vi "LogicalSort.vi"(2 "Input Array":cluster{"date/time string":string, i32}[](array[cluster])=[{"date/time string"="NI_ChannelLength", 0}, {"date/time string"="NI_DataType", 1}, {"date/time string"="name", 2}, {"date/time string"="NI_Scaling_Status", 3}, {"date/time string"="NI_Number_Of_Scales", 4}, {"date/time string"="NI_Scale[1]_Scale_Type", 5}, {"date/time string"="NI_Scale[1]_Linear_Slope", 6}, {"date/time string"="NI_Scale[1]_Linear_Y_Intercept", 7}, {"date/time string"="NI_Scale[1]_Linear_Input_Source", 8}, {"date/time string"="NI_Scale[3]_Scale_Type", 9}, {"date/time string"="NI_Scale[3]_Linear_Slope", 10}, {"date/time string"="NI_Scale[3]_Linear_Y_Intercept", 11}, {"date/time string"="NI_Scale[3]_Linear_Input_Source", 12}, {"date/time string"="NI_Scale[4]_Scale_Type", 13}, {"date/time string"="NI_Scale[4]_Subtract_Left_Operand_Input_Source", 14}, {"date/time string"="NI_Scale[4]_Subtract_Right_Operand_Input_Source", 15}, {"date/time string"="NI_Scale[5]_Scale_Type", 16}, {"date/time string"="NI_Scale[5]_Linear_Slope", 17}, {"date/time string"="NI_Scale[5]_Linear_Y_Intercept", 18}, {"date/time string"="NI_Scale[5]_Linear_Input_Source", 19}, {"date/time string"="NI_Scale[7]_Scale_Type", 20}, {"date/time string"="NI_Scale[7]_Linear_Slope", 21}, {"date/time string"="NI_Scale[7]_Linear_Y_Intercept", 22}, {"date/time string"="NI_Scale[7]_Linear_Input_Source", 23}, {"date/time string"="NI_Scale[9]_Scale_Type", 24}, {"date/time string"="NI_Scale[9]_Linear_Slope", 25}, {"date/time string"="NI_Scale[9]_Linear_Y_Intercept", 26}, {"date/time string"="NI_Scale[9]_Linear_Input_Source", 27}, {"date/time string"="NI_Scale[10]_Scale_Type", 28}, {"date/time string"="NI_Scale[10]_Subtract_Left_Operand_Input_Source", 29}, {"date/time string"="NI_Scale[10]_Subtract_Right_Operand_Input_Source", 30}, {"date/time string"="NI_Scale[11]_Scale_Type", 31}, {"date/time string"="NI_Scale[11]_Table_Scaled_Values_Size", 32}, {"date/time string"="NI_Scale[11]_Table_Scaled_Values[0]", 33}, {"date/time string"="NI_Scale[11]_Table_Scaled_Values[1]", 34}, {"date/time string"="NI_Scale[11]_Table_Scaled_Values[2]", 35}, {"date/time string"="NI_Scale[11]_Table_Scaled_Values[3]", 36}, {"date/time string"="NI_Scale[11]_Table_Scaled_Values[4]", 37}, {"date/time string"="NI_Scale[11]_Table_Scaled_Values[5]", 38}, {"date/time string"="NI_Scale[11]_Table_Scaled_Values[6]", 39}, {"date/time string"="NI_Scale[11]_Table_Scaled_Values[7]", 40}, {"date/time string"="NI_Scale[11]_Table_Scaled_Values[8]", 41}, {"date/time string"="NI_Scale[11]_Table_Scaled_Values[9]", 42}, {"date/time string"="NI_Scale[11]_Table_Scaled_Values[10]", 43}, {"date/time string"="NI_Scale[11]_Table_Scaled_Values[11]", 44}, {"date/time string"="NI_Scale[11]_Table_Scaled_Values[12]", 45}, {"date/time string"="NI_Scale[11]_Table_Scaled_Values[13]", 46}, {"date/time string"="NI_Scale[11]_Table_Scaled_Values[14]", 47}, {"date/time string"="NI_Scale[11]_Table_Scaled_Values[15]", 48}, {"date/time string"="NI_Scale[11]_Table_Scaled_Values[16]", 49}, {"date/time string"="NI_Scale[11]_Table_Scaled_Values[17]", 50}, {"date/time string"="NI_Scale[11]_Table_Scaled_Values[18]", 51}, {"date/time string"="NI_Scale[11]_Table_Scaled_Values[19]", 52}, {"date/time string"="NI_Scale[11]_Table_Scaled_Values[20]", 53}, {"date/time string"="NI_Scale[11]_Table_Scaled_Values[21]", 54}, {"date/time string"="NI_Scale[11]_Table_Scaled_Values[22]", 55}, {"date/time string"="NI_Scale[11]_Table_Scaled_Values[23]", 56}, {"date/time string"="NI_Scale[11]_Table_Scaled_Values[24]", 57}, {"date/time string"="NI_Scale[11]_Table_Scaled_Values[25]", 58}, {"date/time string"="NI_Scale[11]_Table_Scaled_Values[26]", 59}, {"date/time string"="NI_Scale[11]_Table_Scaled_Values[27]", 60}, {"date/time string"="NI_Scale[11]_Table_Scaled_Values[28]", 61}, {"date/time string"="NI_Scale[11]_Table_Scaled_Values[29]", 62}, {"date/time string"="NI_Scale[11]_Table_Scaled_Values[30]", 63}, {"date/time string"="NI_Scale[11]_Table_Scaled_Values[31]", 64}, {"date/time string"="NI_Scale[11]_Table_Scaled_Values[32]", 65}, {"date/time string"="NI_Scale[11]_Table_Scaled_Values[33]", 66}, {"date/time string"="NI_Scale[11]_Table_Scaled_Values[34]", 67}, {"date/time string"="NI_Scale[11]_Table_Scaled_Values[35]", 68}, {"date/time string"="NI_Scale[11]_Table_Scaled_Values[36]", 69}, {"date/time string"="NI_Scale[11]_Table_Scaled_Values[37]", 70}, {"date/time string"="NI_Scale[11]_Table_Scaled_Values[38]", 71}, {"date/time string"="NI_Scale[11]_Table_Scaled_Values[39]", 72}, {"date/time string"="NI_Scale[11]_Table_Scaled_Values[40]", 73}, {"date/time string"="NI_Scale[11]_Table_Scaled_Values[41]", 74}, {"date/time string"="NI_Scale[11]_Table_Scaled_Values[42]", 75}, {"date/time string"="NI_Scale[11]_Table_Scaled_Values[43]", 76}, {"date/time string"="NI_Scale[11]_Table_Scaled_Values[44]", 77}, {"date/time string"="NI_Scale[11]_Table_Scaled_Values[45]", 78}, {"date/time string"="NI_Scale[11]_Table_Scaled_Values[46]", 79}, {"date/time string"="NI_Scale[11]_Table_Scaled_Values[47]", 80}, {"date/time string"="NI_Scale[11]_Table_Scaled_Values[48]", 81}, {"date/time string"="NI_Scale[11]_Table_Scaled_Values[49]", 82}, {"date/time string"="NI_Scale[11]_Table_Scaled_Values[50]", 83}, {"date/time string"="NI_Scale[11]_Table_Scaled_Values[51]", 84}, {"date/time string"="NI_Scale[11]_Table_Scaled_Values[52]", 85}, {"date/time string"="NI_Scale[11]_Table_Scaled_Values[53]", 86}, {"date/time string"="NI_Scale[11]_Table_Scaled_Values[54]", 87}, {"date/time string"="NI_Scale[11]_Table_Scaled_Values[55]", 88}, {"date/time string"="NI_Scale[11]_Table_Scaled_Values[56]", 89}, {"date/time string"="NI_Scale[11]_Table_Scaled_Values[57]", 90}, {"date/time string"="NI_Scale[11]_Table_Scaled_Values[58]", 91}, {"date/time string"="NI_Scale[11]_Table_Scaled_Values[59]", 92}, {"date/time string"="NI_Scale[11]_Table_Scaled_Values[60]", 93}, {"date/time string"="NI_Scale[11]_Table_Scaled_Values[61]", 94}, {"date/time string"="NI_Scale[11]_Table_Scaled_Values[62]", 95}, {"date/time string"="NI_Scale[11]_Table_Scaled_Values[63]", 96}, {"date/time string"="NI_Scale[11]_Table_Scaled_Values[64]", 97}, {"date/time string"="NI_Scale[11]_Table_Scaled_Values[65]", 98}, {"date/time string"="NI_Scale[11]_Table_Scaled_Values[66]", 99}, {"date/time string"="NI_Scale[11]_Table_Scaled_Values[67]", 100}, {"date/time string"="NI_Scale[11]_Table_Scaled_Values[68]", 101}, {"date/time string"="NI_Scale[11]_Table_Scaled_Values[69]", 102}, {"date/time string"="NI_Scale[11]_Table_Scaled_Values[70]", 103}, {"date/time string"="NI_Scale[11]_Table_Scaled_Values[71]", 104}, {"date/time string"="NI_Scale[11]_Table_Scaled_Values[72]", 105}, {"date/time string"="NI_Scale[11]_Table_Scaled_Values[73]", 106}, {"date/time string"="NI_Scale[11]_Table_Scaled_Values[74]", 107}, {"date/time string"="NI_Scale[11]_Table_Scaled_Values[75]", 108}, {"date/time string"="NI_Scale[11]_Table_Scaled_Values[76]", 109}, {"date/time string"="NI_Scale[11]_Table_Scaled_Values[77]", 110}, {"date/time string"="NI_Scale[11]_Table_Scaled_Values[78]", 111}, {"date/time string"="NI_Scale[11]_Table_Scaled_Values[79]", 112}, {"date/time string"="NI_Scale[11]_Table_Scaled_Values[80]", 113}, {"date/time string"="NI_Scale[11]_Table_Scaled_Values[81]", 114}, {"date/time string"="NI_Scale[11]_Table_Scaled_Values[82]", 115}, {"date/time string"="NI_Scale[11]_Table_Scaled_Values[83]", 116}, {"date/time string"="NI_Scale[11]_Table_Scaled_Values[84]", 117}, {"date/time string"="NI_Scale[11]_Table_Scaled_Values[85]", 118}, {"date/time string"="NI_Scale[11]_Table_Scaled_Values[86]", 119}, {"date/time string"="NI_Scale[11]_Table_Scaled_Values[87]", 120}, {"date/time string"="NI_Scale[11]_Table_Scaled_Values[88]", 121}, {"date/time string"="NI_Scale[11]_Table_Scaled_Values[89]", 122}, {"date/time string"="NI_Scale[11]_Table_Scaled_Values[90]", 123}, {"date/time string"="NI_Scale[11]_Table_Scaled_Values[91]", 124}, {"date/time string"="NI_Scale[11]_Table_Scaled_Values[92]", 125}, {"date/time string"="NI_Scale[11]_Table_Scaled_Values[93]", 126}, {"date/time string"="NI_Scale[11]_Table_Scaled_Values[94]", 127}, {"date/time string"="NI_Scale[11]_Table_Scaled_Values[95]", 128}, {"date/time string"="NI_Scale[11]_Table_Scaled_Values[96]", 129}, {"date/time string"="NI_Scale[11]_Table_Scaled_Values[97]", 130}, {"date/time string"="NI_Scale[11]_Table_Scaled_Values[98]", 131}, {"date/time string"="NI_Scale[11]_Table_Scaled_Values[99]", 132}, {"date/time string"="NI_Scale[11]_Table_Scaled_Values[100]", 133}, {"date/time string"="NI_Scale[11]_Table_Scaled_Values[101]", 134}, {"date/time string"="NI_Scale[11]_Table_Scaled_Values[102]", 135}, {"date/time string"="NI_Scale[11]_Table_Scaled_Values[103]", 136}, {"date/time string"="NI_Scale[11]_Table_Scaled_Values[104]", 137}, {"date/time string"="NI_Scale[11]_Table_Scaled_Values[105]", 138}, {"date/time string"="NI_Scale[11]_Table_Scaled_Values[106]", 139}, {"date/time string"="NI_Scale[11]_Table_Scaled_Values[107]", 140}, {"date/time string"="NI_Scale[11]_Table_Scaled_Values[108]", 141}, {"date/time string"="NI_Scale[11]_Table_Scaled_Values[109]", 142}, {"date/time string"="NI_Scale[11]_Table_Scaled_Values[110]", 143}, {"date/time string"="NI_Scale[11]_Table_Scaled_Values[111]", 144}, {"date/time string"="NI_Scale[11]_Table_Scaled_Values[112]", 145}, {"date/time string"="NI_Scale[11]_Table_Scaled_Values[113]", 146}, {"date/time string"="NI_Scale[11]_Table_Scaled_Values[114]", 147}, {"date/time string"="NI_Scale[11]_Table_Scaled_Values[115]", 148}, {"date/time string"="NI_Scale[11]_Table_Scaled_Values[116]", 149}, {"date/time string"="NI_Scale[11]_Table_Scaled_Values[117]", 150}, {"date/time string"="NI_Scale[11]_Table_Scaled_Values[118]", 151}, {"date/time string"="NI_Scale[11]_Table_Scaled_Values[119]", 152}, {"date/time string"="NI_Scale[11]_Table_Scaled_Values[120]", 153}, {"date/time string"="NI_Scale[11]_Table_Scaled_Values[121]", 154}, {"date/time string"="NI_Scale[11]_Table_Scaled_Values[122]", 155}, {"date/time string"="NI_Scale[11]_Table_Scaled_Values[123]", 156}, {"date/time string"="NI_Scale[11]_Table_Scaled_Values[124]", 157}, {"date/time string"="NI_Scale[11]_Table_Scaled_Values[125]", 158}, {"date/time string"="NI_Scale[11]_Table_Scaled_Values[126]", 159}, {"date/time string"="NI_Scale[11]_Table_Scaled_Values[127]", 160}, {"date/time string"="NI_Scale[11]_Table_Scaled_Values[128]", 161}, {"date/time string"="NI_Scale[11]_Table_Scaled_Values[129]", 162}, {"date/time string"="NI_Scale[11]_Table_Scaled_Values[130]", 163}, {"date/time string"="NI_Scale[11]_Table_Scaled_Values[131]", 164}, {"date/time string"="NI_Scale[11]_Table_Scaled_Values[132]", 165}, {"date/time string"="NI_Scale[11]_Table_Scaled_Values[133]", 166}, {"date/time string"="NI_Scale[11]_Table_Scaled_Values[134]", 167}, {"date/time string"="NI_Scale[11]_Table_Scaled_Values[135]", 168}, {"date/time string"="NI_Scale[11]_Table_Scaled_Values[136]", 169}, {"date/time string"="NI_Scale[11]_Table_Scaled_Values[137]", 170}, {"date/time string"="NI_Scale[11]_Table_Scaled_Values[138]", 171}, {"date/time string"="NI_Scale[11]_Table_Scaled_Values[139]", 172}, {"date/time string"="NI_Scale[11]_Table_Scaled_Values[140]", 173}, {"date/time string"="NI_Scale[11]_Table_Scaled_Values[141]", 174}, {"date/time string"="NI_Scale[11]_Table_Scaled_Values[142]", 175}, {"date/time string"="NI_Scale[11]_Table_Scaled_Values[143]", 176}, {"date/time string"="NI_Scale[11]_Table_Scaled_Values[144]", 177}, {"date/time string"="NI_Scale[11]_Table_Scaled_Values[145]", 178}, {"date/time string"="NI_Scale[11]_Table_Scaled_Values[146]", 179}, {"date/time string"="NI_Scale[11]_Table_Scaled_Values[147]", 180}, {"date/time string"="NI_Scale[11]_Table_Scaled_Values[148]", 181}, {"date/time string"="NI_Scale[11]_Table_Scaled_Values[149]", 182}, {"date/time string"="NI_Scale[11]_Table_Scaled_Values[150]", 183}, {"date/time string"="NI_Scale[11]_Table_Scaled_Values[151]", 184}, {"date/time string"="NI_Scale[11]_Table_Scaled_Values[152]", 185}, {"date/time string"="NI_Scale[11]_Table_Scaled_Values[153]", 186}, {"date/time string"="NI_Scale[11]_Table_Scaled_Values[154]", 187}, {"date/time string"="NI_Scale[11]_Table_Scaled_Values[155]", 188}, {"date/time string"="NI_Scale[11]_Table_Scaled_Values[156]", 189}, {"date/time string"="NI_Scale[11]_Table_Scaled_Values[157]", 190}, {"date/time string"="NI_Scale[11]_Table_Scaled_Values[158]", 191}, {"date/time string"="NI_Scale[11]_Table_Scaled_Values[159]", 192}, {"date/time string"="NI_Scale[11]_Table_Scaled_Values[160]", 193}, {"date/time string"="NI_Scale[11]_Table_Scaled_Values[161]", 194}, {"date/time string"="NI_Scale[11]_Table_Scaled_Values[162]", 195}, {"date/time string"="NI_Scale[11]_Table_Scaled_Values[163]", 196}, {"date/time string"="NI_Scale[11]_Table_Scaled_Values[164]", 197}, {"date/time string"="NI_Scale[11]_Table_Scaled_Values[165]", 198}, {"date/time string"="NI_Scale[11]_Table_Scaled_Values[166]", 199}, {"date/time string"="NI_Scale[11]_Table_Scaled_Values[167]", 200}, {"date/time string"="NI_Scale[11]_Table_Scaled_Values[168]", 201}, {"date/time string"="NI_Scale[11]_Table_Scaled_Values[169]", 202}, {"date/time string"="NI_Scale[11]_Table_Scaled_Values[170]", 203}, {"date/time string"="NI_Scale[11]_Table_Scaled_Values[171]", 204}, {"date/time string"="NI_Scale[11]_Table_Scaled_Values[172]", 205}, {"date/time string"="NI_Scale[11]_Table_Scaled_Values[173]", 206}, {"date/time string"="NI_Scale[11]_Table_Scaled_Values[174]", 207}, {"date/time string"="NI_Scale[11]_Table_Scaled_Values[175]", 208}, {"date/time string"="NI_Scale[11]_Table_Scaled_Values[176]", 209}, {"date/time string"="NI_Scale[11]_Table_Scaled_Values[177]", 210}, {"date/time string"="NI_Scale[11]_Table_Scaled_Values[178]", 211}, {"date/time string"="NI_Scale[11]_Table_Scaled_Values[179]", 212}, {"date/time string"="NI_Scale[11]_Table_Scaled_Values[180]", 213}, {"date/time string"="NI_Scale[11]_Table_Scaled_Values[181]", 214}, {"date/time string"="NI_Scale[11]_Table_Scaled_Values[182]", 215}, {"date/time string"="NI_Scale[11]_Table_Scaled_Values[183]", 216}, {"date/time string"="NI_Scale[11]_Table_Scaled_Values[184]", 217}, {"date/time string"="NI_Scale[11]_Table_Scaled_Values[185]", 218}, {"date/time string"="NI_Scale[11]_Table_Scaled_Values[186]", 219}, {"date/time string"="NI_Scale[11]_Table_Scaled_Values[187]", 220}, {"date/time string"="NI_Scale[11]_Table_Scaled_Values[188]", 221}, {"date/time string"="NI_Scale[11]_Table_Scaled_Values[189]", 222}, {"date/time string"="NI_Scale[11]_Table_Scaled_Values[190]", 223}, {"date/time string"="NI_Scale[11]_Table_Scaled_Values[191]", 224}, {"date/time string"="NI_Scale[11]_Table_Scaled_Values[192]", 225}, {"date/time string"="NI_Scale[11]_Table_Scaled_Values[193]", 226}, {"date/time string"="NI_Scale[11]_Table_Scaled_Values[194]", 227}, {"date/time string"="NI_Scale[11]_Table_Scaled_Values[195]", 228}, {"date/time string"="NI_Scale[11]_Table_Scaled_Values[196]", 229}, {"date/time string"="NI_Scale[11]_Table_Scaled_Values[197]", 230}, {"date/time string"="NI_Scale[11]_Table_Scaled_Values[198]", 231}, {"date/time string"="NI_Scale[11]_Table_Scaled_Values[199]", 232}, {"date/time string"="NI_Scale[11]_Table_Scaled_Values[200]", 233}, {"date/time string"="NI_Scale[11]_Table_Scaled_Values[201]", 234}, {"date/time string"="NI_Scale[11]_Table_Scaled_Values[202]", 235}, {"date/time string"="NI_Scale[11]_Table_Scaled_Values[203]", 236}, {"date/time string"="NI_Scale[11]_Table_Scaled_Values[204]", 237}, {"date/time string"="NI_Scale[11]_Table_Scaled_Values[205]", 238}, {"date/time string"="NI_Scale[11]_Table_Pre_Scaled_Values_Size", 239}, {"date/time string"="NI_Scale[11]_Table_Pre_Scaled_Values[0]", 240}, {"date/time string"="NI_Scale[11]_Table_Pre_Scaled_Values[1]", 241}, {"date/time string"="NI_Scale[11]_Table_Pre_Scaled_Values[2]", 242}, {"date/time string"="NI_Scale[11]_Table_Pre_Scaled_Values[3]", 243}, {"date/time string"="NI_Scale[11]_Table_Pre_Scaled_Values[4]", 244}, {"date/time string"="NI_Scale[11]_Table_Pre_Scaled_Values[5]", 245}, {"date/time string"="NI_Scale[11]_Table_Pre_Scaled_Values[6]", 246}, {"date/time string"="NI_Scale[11]_Table_Pre_Scaled_Values[7]", 247}, {"date/time string"="NI_Scale[11]_Table_Pre_Scaled_Values[8]", 248}, {"date/time string"="NI_Scale[11]_Table_Pre_Scaled_Values[9]", 249}, {"date/time string"="NI_Scale[11]_Table_Pre_Scaled_Values[10]", 250}, {"date/time string"="NI_Scale[11]_Table_Pre_Scaled_Values[11]", 251}, {"date/time string"="NI_Scale[11]_Table_Pre_Scaled_Values[12]", 252}, {"date/time string"="NI_Scale[11]_Table_Pre_Scaled_Values[13]", 253}, {"date/time string"="NI_Scale[11]_Table_Pre_Scaled_Values[14]", 254}, {"date/time string"="NI_Scale[11]_Table_Pre_Scaled_Values[15]", 255}, {"date/time string"="NI_Scale[11]_Table_Pre_Scaled_Values[16]", 256}, {"date/time string"="NI_Scale[11]_Table_Pre_Scaled_Values[17]", 257}, {"date/time string"="NI_Scale[11]_Table_Pre_Scaled_Values[18]", 258}, {"date/time string"="NI_Scale[11]_Table_Pre_Scaled_Values[19]", 259}, {"date/time string"="NI_Scale[11]_Table_Pre_Scaled_Values[20]", 260}, {"date/time string"="NI_Scale[11]_Table_Pre_Scaled_Values[21]", 261}, {"date/time string"="NI_Scale[11]_Table_Pre_Scaled_Values[22]", 262}, {"date/time string"="NI_Scale[11]_Table_Pre_Scaled_Values[23]", 263}, {"date/time string"="NI_Scale[11]_Table_Pre_Scaled_Values[24]", 264}, {"date/time string"="NI_Scale[11]_Table_Pre_Scaled_Values[25]", 265}, {"date/time string"="NI_Scale[11]_Table_Pre_Scaled_Values[26]", 266}, {"date/time string"="NI_Scale[11]_Table_Pre_Scaled_Values[27]", 267}, {"date/time string"="NI_Scale[11]_Table_Pre_Scaled_Values[28]", 268}, {"date/time string"="NI_Scale[11]_Table_Pre_Scaled_Values[29]", 269}, {"date/time string"="NI_Scale[11]_Table_Pre_Scaled_Values[30]", 270}, {"date/time string"="NI_Scale[11]_Table_Pre_Scaled_Values[31]", 271}, {"date/time string"="NI_Scale[11]_Table_Pre_Scaled_Values[32]", 272}, {"date/time string"="NI_Scale[11]_Table_Pre_Scaled_Values[33]", 273}, {"date/time string"="NI_Scale[11]_Table_Pre_Scaled_Values[34]", 274}, {"date/time string"="NI_Scale[11]_Table_Pre_Scaled_Values[35]", 275}, {"date/time string"="NI_Scale[11]_Table_Pre_Scaled_Values[36]", 276}, {"date/time string"="NI_Scale[11]_Table_Pre_Scaled_Values[37]", 277}, {"date/time string"="NI_Scale[11]_Table_Pre_Scaled_Values[38]", 278}, {"date/time string"="NI_Scale[11]_Table_Pre_Scaled_Values[39]", 279}, {"date/time string"="NI_Scale[11]_Table_Pre_Scaled_Values[40]", 280}, {"date/time string"="NI_Scale[11]_Table_Pre_Scaled_Values[41]", 281}, {"date/time string"="NI_Scale[11]_Table_Pre_Scaled_Values[42]", 282}, {"date/time string"="NI_Scale[11]_Table_Pre_Scaled_Values[43]", 283}, {"date/time string"="NI_Scale[11]_Table_Pre_Scaled_Values[44]", 284}, {"date/time string"="NI_Scale[11]_Table_Pre_Scaled_Values[45]", 285}, {"date/time string"="NI_Scale[11]_Table_Pre_Scaled_Values[46]", 286}, {"date/time string"="NI_Scale[11]_Table_Pre_Scaled_Values[47]", 287}, {"date/time string"="NI_Scale[11]_Table_Pre_Scaled_Values[48]", 288}, {"date/time string"="NI_Scale[11]_Table_Pre_Scaled_Values[49]", 289}, {"date/time string"="NI_Scale[11]_Table_Pre_Scaled_Values[50]", 290}, {"date/time string"="NI_Scale[11]_Table_Pre_Scaled_Values[51]", 291}, {"date/time string"="NI_Scale[11]_Table_Pre_Scaled_Values[52]", 292}, {"date/time string"="NI_Scale[11]_Table_Pre_Scaled_Values[53]", 293}, {"date/time string"="NI_Scale[11]_Table_Pre_Scaled_Values[54]", 294}, {"date/time string"="NI_Scale[11]_Table_Pre_Scaled_Values[55]", 295}, {"date/time string"="NI_Scale[11]_Table_Pre_Scaled_Values[56]", 296}, {"date/time string"="NI_Scale[11]_Table_Pre_Scaled_Values[57]", 297}, {"date/time string"="NI_Scale[11]_Table_Pre_Scaled_Values[58]", 298}, {"date/time string"="NI_Scale[11]_Table_Pre_Scaled_Values[59]", 299}, {"date/time string"="NI_Scale[11]_Table_Pre_Scaled_Values[60]", 300}, {"date/time string"="NI_Scale[11]_Table_Pre_Scaled_Values[61]", 301}, {"date/time string"="NI_Scale[11]_Table_Pre_Scaled_Values[62]", 302}, {"date/time string"="NI_Scale[11]_Table_Pre_Scaled_Values[63]", 303}, {"date/time string"="NI_Scale[11]_Table_Pre_Scaled_Values[64]", 304}, {"date/time string"="NI_Scale[11]_Table_Pre_Scaled_Values[65]", 305}, {"date/time string"="NI_Scale[11]_Table_Pre_Scaled_Values[66]", 306}, {"date/time string"="NI_Scale[11]_Table_Pre_Scaled_Values[67]", 307}, {"date/time string"="NI_Scale[11]_Table_Pre_Scaled_Values[68]", 308}, {"date/time string"="NI_Scale[11]_Table_Pre_Scaled_Values[69]", 309}, {"date/time string"="NI_Scale[11]_Table_Pre_Scaled_Values[70]", 310}, {"date/time string"="NI_Scale[11]_Table_Pre_Scaled_Values[71]", 311}, {"date/time string"="NI_Scale[11]_Table_Pre_Scaled_Values[72]", 312}, {"date/time string"="NI_Scale[11]_Table_Pre_Scaled_Values[73]", 313}, {"date/time string"="NI_Scale[11]_Table_Pre_Scaled_Values[74]", 314}, {"date/time string"="NI_Scale[11]_Table_Pre_Scaled_Values[75]", 315}, {"date/time string"="NI_Scale[11]_Table_Pre_Scaled_Values[76]", 316}, {"date/time string"="NI_Scale[11]_Table_Pre_Scaled_Values[77]", 317}, {"date/time string"="NI_Scale[11]_Table_Pre_Scaled_Values[78]", 318}, {"date/time string"="NI_Scale[11]_Table_Pre_Scaled_Values[79]", 319}, {"date/time string"="NI_Scale[11]_Table_Pre_Scaled_Values[80]", 320}, {"date/time string"="NI_Scale[11]_Table_Pre_Scaled_Values[81]", 321}, {"date/time string"="NI_Scale[11]_Table_Pre_Scaled_Values[82]", 322}, {"date/time string"="NI_Scale[11]_Table_Pre_Scaled_Values[83]", 323}, {"date/time string"="NI_Scale[11]_Table_Pre_Scaled_Values[84]", 324}, {"date/time string"="NI_Scale[11]_Table_Pre_Scaled_Values[85]", 325}, {"date/time string"="NI_Scale[11]_Table_Pre_Scaled_Values[86]", 326}, {"date/time string"="NI_Scale[11]_Table_Pre_Scaled_Values[87]", 327}, {"date/time string"="NI_Scale[11]_Table_Pre_Scaled_Values[88]", 328}, {"date/time string"="NI_Scale[11]_Table_Pre_Scaled_Values[89]", 329}, {"date/time string"="NI_Scale[11]_Table_Pre_Scaled_Values[90]", 330}, {"date/time string"="NI_Scale[11]_Table_Pre_Scaled_Values[91]", 331}, {"date/time string"="NI_Scale[11]_Table_Pre_Scaled_Values[92]", 332}, {"date/time string"="NI_Scale[11]_Table_Pre_Scaled_Values[93]", 333}, {"date/time string"="NI_Scale[11]_Table_Pre_Scaled_Values[94]", 334}, {"date/time string"="NI_Scale[11]_Table_Pre_Scaled_Values[95]", 335}, {"date/time string"="NI_Scale[11]_Table_Pre_Scaled_Values[96]", 336}, {"date/time string"="NI_Scale[11]_Table_Pre_Scaled_Values[97]", 337}, {"date/time string"="NI_Scale[11]_Table_Pre_Scaled_Values[98]", 338}, {"date/time string"="NI_Scale[11]_Table_Pre_Scaled_Values[99]", 339}, {"date/time string"="NI_Scale[11]_Table_Pre_Scaled_Values[100]", 340}, {"date/time string"="NI_Scale[11]_Table_Pre_Scaled_Values[101]", 341}, {"date/time string"="NI_Scale[11]_Table_Pre_Scaled_Values[102]", 342}, {"date/time string"="NI_Scale[11]_Table_Pre_Scaled_Values[103]", 343}, {"date/time string"="NI_Scale[11]_Table_Pre_Scaled_Values[104]", 344}, {"date/time string"="NI_Scale[11]_Table_Pre_Scaled_Values[105]", 345}, {"date/time string"="NI_Scale[11]_Table_Pre_Scaled_Values[106]", 346}, {"date/time string"="NI_Scale[11]_Table_Pre_Scaled_Values[107]", 347}, {"date/time string"="NI_Scale[11]_Table_Pre_Scaled_Values[108]", 348}, {"date/time string"="NI_Scale[11]_Table_Pre_Scaled_Values[109]", 349}, {"date/time string"="NI_Scale[11]_Table_Pre_Scaled_Values[110]", 350}, {"date/time string"="NI_Scale[11]_Table_Pre_Scaled_Values[111]", 351}, {"date/time string"="NI_Scale[11]_Table_Pre_Scaled_Values[112]", 352}, {"date/time string"="NI_Scale[11]_Table_Pre_Scaled_Values[113]", 353}, {"date/time string"="NI_Scale[11]_Table_Pre_Scaled_Values[114]", 354}, {"date/time string"="NI_Scale[11]_Table_Pre_Scaled_Values[115]", 355}, {"date/time string"="NI_Scale[11]_Table_Pre_Scaled_Values[116]", 356}, {"date/time string"="NI_Scale[11]_Table_Pre_Scaled_Values[117]", 357}, {"date/time string"="NI_Scale[11]_Table_Pre_Scaled_Values[118]", 358}, {"date/time string"="NI_Scale[11]_Table_Pre_Scaled_Values[119]", 359}, {"date/time string"="NI_Scale[11]_Table_Pre_Scaled_Values[120]", 360}, {"date/time string"="NI_Scale[11]_Table_Pre_Scaled_Values[121]", 361}, {"date/time string"="NI_Scale[11]_Table_Pre_Scaled_Values[122]", 362}, {"date/time string"="NI_Scale[11]_Table_Pre_Scaled_Values[123]", 363}, {"date/time string"="NI_Scale[11]_Table_Pre_Scaled_Values[124]", 364}, {"date/time string"="NI_Scale[11]_Table_Pre_Scaled_Values[125]", 365}, {"date/time string"="NI_Scale[11]_Table_Pre_Scaled_Values[126]", 366}, {"date/time string"="NI_Scale[11]_Table_Pre_Scaled_Values[127]", 367}, {"date/time string"="NI_Scale[11]_Table_Pre_Scaled_Values[128]", 368}, {"date/time string"="NI_Scale[11]_Table_Pre_Scaled_Values[129]", 369}, {"date/time string"="NI_Scale[11]_Table_Pre_Scaled_Values[130]", 370}, {"date/time string"="NI_Scale[11]_Table_Pre_Scaled_Values[131]", 371}, {"date/time string"="NI_Scale[11]_Table_Pre_Scaled_Values[132]", 372}, {"date/time string"="NI_Scale[11]_Table_Pre_Scaled_Values[133]", 373}, {"date/time string"="NI_Scale[11]_Table_Pre_Scaled_Values[134]", 374}, {"date/time string"="NI_Scale[11]_Table_Pre_Scaled_Values[135]", 375}, {"date/time string"="NI_Scale[11]_Table_Pre_Scaled_Values[136]", 376}, {"date/time string"="NI_Scale[11]_Table_Pre_Scaled_Values[137]", 377}, {"date/time string"="NI_Scale[11]_Table_Pre_Scaled_Values[138]", 378}, {"date/time string"="NI_Scale[11]_Table_Pre_Scaled_Values[139]", 379}, {"date/time string"="NI_Scale[11]_Table_Pre_Scaled_Values[140]", 380}, {"date/time string"="NI_Scale[11]_Table_Pre_Scaled_Values[141]", 381}, {"date/time string"="NI_Scale[11]_Table_Pre_Scaled_Values[142]", 382}, {"date/time string"="NI_Scale[11]_Table_Pre_Scaled_Values[143]", 383}, {"date/time string"="NI_Scale[11]_Table_Pre_Scaled_Values[144]", 384}, {"date/time string"="NI_Scale[11]_Table_Pre_Scaled_Values[145]", 385}, {"date/time string"="NI_Scale[11]_Table_Pre_Scaled_Values[146]", 386}, {"date/time string"="NI_Scale[11]_Table_Pre_Scaled_Values[147]", 387}, {"date/time string"="NI_Scale[11]_Table_Pre_Scaled_Values[148]", 388}, {"date/time string"="NI_Scale[11]_Table_Pre_Scaled_Values[149]", 389}, {"date/time string"="NI_Scale[11]_Table_Pre_Scaled_Values[150]", 390}, {"date/time string"="NI_Scale[11]_Table_Pre_Scaled_Values[151]", 391}, {"date/time string"="NI_Scale[11]_Table_Pre_Scaled_Values[152]", 392}, {"date/time string"="NI_Scale[11]_Table_Pre_Scaled_Values[153]", 393}, {"date/time string"="NI_Scale[11]_Table_Pre_Scaled_Values[154]", 394}, {"date/time string"="NI_Scale[11]_Table_Pre_Scaled_Values[155]", 395}, {"date/time string"="NI_Scale[11]_Table_Pre_Scaled_Values[156]", 396}, {"date/time string"="NI_Scale[11]_Table_Pre_Scaled_Values[157]", 397}, {"date/time string"="NI_Scale[11]_Table_Pre_Scaled_Values[158]", 398}, {"date/time string"="NI_Scale[11]_Table_Pre_Scaled_Values[159]", 399}, {"date/time string"="NI_Scale[11]_Table_Pre_Scaled_Values[160]", 400}, {"date/time string"="NI_Scale[11]_Table_Pre_Scaled_Values[161]", 401}, {"date/time string"="NI_Scale[11]_Table_Pre_Scaled_Values[162]", 402}, {"date/time string"="NI_Scale[11]_Table_Pre_Scaled_Values[163]", 403}, {"date/time string"="NI_Scale[11]_Table_Pre_Scaled_Values[164]", 404}, {"date/time string"="NI_Scale[11]_Table_Pre_Scaled_Values[165]", 405}, {"date/time string"="NI_Scale[11]_Table_Pre_Scaled_Values[166]", 406}, {"date/time string"="NI_Scale[11]_Table_Pre_Scaled_Values[167]", 407}, {"date/time string"="NI_Scale[11]_Table_Pre_Scaled_Values[168]", 408}, {"date/time string"="NI_Scale[11]_Table_Pre_Scaled_Values[169]", 409}, {"date/time string"="NI_Scale[11]_Table_Pre_Scaled_Values[170]", 410}, {"date/time string"="NI_Scale[11]_Table_Pre_Scaled_Values[171]", 411}, {"date/time string"="NI_Scale[11]_Table_Pre_Scaled_Values[172]", 412}, {"date/time string"="NI_Scale[11]_Table_Pre_Scaled_Values[173]", 413}, {"date/time string"="NI_Scale[11]_Table_Pre_Scaled_Values[174]", 414}, {"date/time string"="NI_Scale[11]_Table_Pre_Scaled_Values[175]", 415}, {"date/time string"="NI_Scale[11]_Table_Pre_Scaled_Values[176]", 416}, {"date/time string"="NI_Scale[11]_Table_Pre_Scaled_Values[177]", 417}, {"date/time string"="NI_Scale[11]_Table_Pre_Scaled_Values[178]", 418}, {"date/time string"="NI_Scale[11]_Table_Pre_Scaled_Values[179]", 419}, {"date/time string"="NI_Scale[11]_Table_Pre_Scaled_Values[180]", 420}, {"date/time string"="NI_Scale[11]_Table_Pre_Scaled_Values[181]", 421}, {"date/time string"="NI_Scale[11]_Table_Pre_Scaled_Values[182]", 422}, {"date/time string"="NI_Scale[11]_Table_Pre_Scaled_Values[183]", 423}, {"date/time string"="NI_Scale[11]_Table_Pre_Scaled_Values[184]", 424}, {"date/time string"="NI_Scale[11]_Table_Pre_Scaled_Values[185]", 425}, {"date/time string"="NI_Scale[11]_Table_Pre_Scaled_Values[186]", 426}, {"date/time string"="NI_Scale[11]_Table_Pre_Scaled_Values[187]", 427}, {"date/time string"="NI_Scale[11]_Table_Pre_Scaled_Values[188]", 428}, {"date/time string"="NI_Scale[11]_Table_Pre_Scaled_Values[189]", 429}, {"date/time string"="NI_Scale[11]_Table_Pre_Scaled_Values[190]", 430}, {"date/time string"="NI_Scale[11]_Table_Pre_Scaled_Values[191]", 431}, {"date/time string"="NI_Scale[11]_Table_Pre_Scaled_Values[192]", 432}, {"date/time string"="NI_Scale[11]_Table_Pre_Scaled_Values[193]", 433}, {"date/time string"="NI_Scale[11]_Table_Pre_Scaled_Values[194]", 434}, {"date/time string"="NI_Scale[11]_Table_Pre_Scaled_Values[195]", 435}, {"date/time string"="NI_Scale[11]_Table_Pre_Scaled_Values[196]", 436}, {"date/time string"="NI_Scale[11]_Table_Pre_Scaled_Values[197]", 437}, {"date/time string"="NI_Scale[11]_Table_Pre_Scaled_Values[198]", 438}, {"date/time string"="NI_Scale[11]_Table_Pre_Scaled_Values[199]", 439}, {"date/time string"="NI_Scale[11]_Table_Pre_Scaled_Values[200]", 440}, {"date/time string"="NI_Scale[11]_Table_Pre_Scaled_Values[201]", 441}, {"date/time string"="NI_Scale[11]_Table_Pre_Scaled_Values[202]", 442}, {"date/time string"="NI_Scale[11]_Table_Pre_Scaled_Values[203]", 443}, {"date/time string"="NI_Scale[11]_Table_Pre_Scaled_Values[204]", 444}, {"date/time string"="NI_Scale[11]_Table_Pre_Scaled_Values[205]", 445}, {"date/time string"="NI_Scale[11]_Table_Input_Source", 446}, {"date/time string"="NI_Scale[12]_Scale_Type", 447}, {"date/time string"="NI_Scale[12]_Linear_Slope", 448}, {"date/time string"="NI_Scale[12]_Linear_Y_Intercept", 449}, {"date/time string"="NI_Scale[12]_Linear_Input_Source", 450}, {"date/time string"="NI_Scale[13]_Scale_Type", 451}, {"date/time string"="NI_Scale[13]_Thermocouple_Thermocouple_Type", 452}, {"date/time string"="NI_Scale[13]_Thermocouple_Scaling_Direction", 453}, {"date/time string"="NI_Scale[13]_Thermocouple_Input_Source", 454}, {"date/time string"="NI_Scale[14]_Scale_Type", 455}, {"date/time string"="NI_Scale[14]_Add_Left_Operand_Input_Source", 456}, {"date/time string"="NI_Scale[14]_Add_Right_Operand_Input_Source", 457}, {"date/time string"="NI_Scale[15]_Scale_Type", 458}, {"date/time string"="NI_Scale[15]_Thermocouple_Thermocouple_Type", 459}, {"date/time string"="NI_Scale[15]_Thermocouple_Scaling_Direction", 460}, {"date/time string"="NI_Scale[15]_Thermocouple_Input_Source", 461}, {"date/time string"="NI_ChannelName", 462}, {"date/time string"="unit_string", 463}, {"date/time string"="NI_UnitDescription", 464}, {"date/time string"="wf_start_time", 465}, {"date/time string"="wf_increment", 466}, {"date/time string"="wf_start_offset", 467}, {"date/time string"="wf_samples", 468}]) -> (7 "Sorted Array":cluster{"date/time string":string, i32}[](array[cluster]))   [LabVIEW 2017]
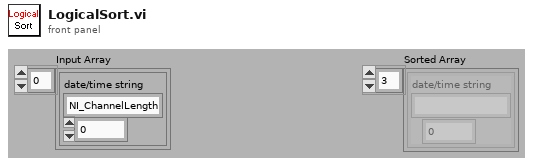
[diagram p1: front panel]
types:
  T1 = cluster{"split str":cluster{"str":string, "num":i32}[], "orig str":string, "index":i32}[]
  T2 = cluster{"split str":cluster{"str":string, "num":i32}[], "orig str":string, "index":i32}
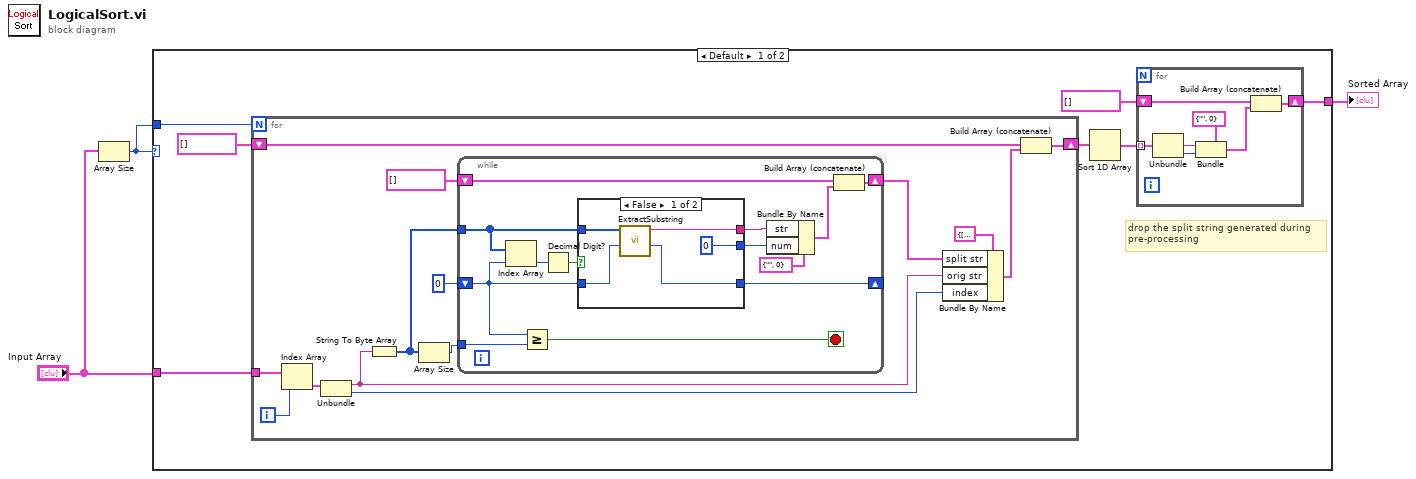
[diagram p0: block diagram]
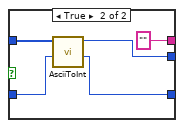
[diagram p2: hidden frame]
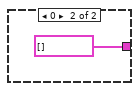
[diagram p3: hidden frame]
diagram:
  n1 = Array Size(array="Input Array") -> (size(s)=w2:i32)
  n2 = case shown="Default" w2 {
    tunnel: [w4 cluster{"date/time string":string, i32}[] [] ("Sorted Array")] -> w1
    tunnel: "Input Array" -> [w10 _]
    tunnel: w2 -> [w9 _]
    frame Default {
      # "drop the split string generated during\npre-processing"
      n3 = for {
        N: w9 -> [_]
        tunnel: w10 -> [w31]
        shift-right: [w25] -> w8
        shift-left: T1 [] ("sorted array") -> [w23]
        i -> [w30]
        n4 = Index Array(array=w31, index=w30) -> (element=w29:cluster{"date/time string":string, i32})
        n5 = Unbundle(w29) -> ("date/time string"=w21:string, w20:i32)
        n6 = String To Byte Array(string=w21) -> (unsigned byte array=w27:u8[])
        n7 = Array Size(array=w27) -> (size(s)=w26:i32)
        n8 = while {
          shift-right: [w40] -> _
          shift-left: 0 ("size(s)") -> [w39]
          tunnel: w27 -> [w43]
          tunnel: w26 -> [w38]
          shift-right: [w34] -> w22
          shift-left: cluster{"str":string, "num":i32}[] [] ("split str") -> [w36]
          stop <- w33 stop-if-true
          n9 = Index Array(array=w43, index=w39) -> (element=w44:u8)
          n10 = Greater Or Equal?(x=w39, y=w38) -> (x >= y?=w33:bool)
          n11 = Decimal Digit?(1:w44) -> (0:w32:bool)
          n12 = case shown="False" w32 {
            tunnel: w43 -> [w47 w54]
            tunnel: [w46 "" ("str")] -> w42
            tunnel: [0 ("value") w50] -> w41
            tunnel: w39 -> [w49 w53]
            tunnel: [w48 w52] -> w40
            frame False {
              n13 = call <vilib>:"ExtractSubstring.vi"("offset"=w49, "string byte array"=w47) -> ("new offset"=w48:i32, "sub string"=w46:string)  [unwired: 8 in]
            }
            frame True {
              n14 = call <vilib>:"AsciiToInt.vi"("offset"=w53, "string byte array"=w54) -> ("new offset"=w52:i32, "value"=w50:i32)  [unwired: 8 in]
            }
          }
          n15 = Bundle By Name(cluster=cluster{"str":string, "num":i32} {"str"="", "num"=0}, "str"=w42, "num"=w41) -> (w35:cluster{"str":string, "num":i32})
          n16 = Build Array (concatenate)(w36, w35) -> (w34:cluster{"str":string, "num":i32}[])
        }
        n17 = Bundle By Name(cluster=T2 {"split str"=[], "orig str"="", "index"=0} ("Cluster"), "split str"=w22, "orig str"=w21, "index"=w20) -> (w19:T2)
        n18 = Build Array (concatenate)(w23, w19) -> (w25:T1)
      }
      n19 = Sort 1D Array(array=w8) -> (sorted array=w5:T1)
      n20 = for {
        tunnel: w5 -> [w17] mode=indexing
        shift-right: [w12] -> w4
        shift-left: cluster{"date/time string":string, i32}[] [] ("Sorted Array") -> [w13]
        n21 = Unbundle(w17) -> ("orig str"=w15:string, "index"=w14:i32)  [unwired: 1 out]
        n22 = Bundle(cluster=cluster{"date/time string":string, i32} {"date/time string"="", 0}, "date/time string"=w15, w14) -> (w11:cluster{"date/time string":string, i32})
        n23 = Build Array (concatenate)(w13, w11) -> (w12:cluster{"date/time string":string, i32}[])
      }
    }
    frame 0 {
    }
  }
  "Sorted Array" <- w1
